vi "Configure Frequency Channel.vi"(7 "Enable Frequency Channel (F:Disable)":bool, 8 "error in (no error)":errorcluster, 9 "Channel Number (1)":i32=1, 10 "Channel Band (2: P-GSM Base)":u16(ring)=2 items=["NADC Base", "NADC Mobile", "P-GSM Base", "P-GSM Mobile", "E-GSM Base", "E-GSM Mobile", "R-GSM Base", "R-GSM Mobile", "DCS Base", "DCS Mobile", "PCS Base", "PCS Mobile", "GSM 450 Base", "GSM 450 Mobile", "GSM 480 Base", "GSM 480 Mobile", "GSM 850 Base", "GSM 850 Mobile", "800MHZ Base", "800MHZ Mobile", "1500MHZ Base", "1500MHZ Mobile", "Tetra Base 390/400", "Tetra Base 420/430", "Tetra Base 460/470", "Tetra Base 915/921", "Tetra Mobile 380/390", "Tetra Mobile 410/420", "Tetra Mobile 450/460", "Tetra Mobile 870/876", "PHS Standard", "DECT Standard"], 11 "VISA resource name":refnum<visa-resource-name>) -> (0 "error out":errorcluster, 3 "VISA resource name out":refnum<visa-resource-name>)   [LabVIEW 2014, in "Agilent PSG MXG Series.lvlib"]
doc: "Configures frequency channel and band.\n\n<B>Notes:</B>\n(1) This VI is valid only in E8247C, E8257C, E8267C, E8257D, E8267D, N5161A, N5162A, N5181A, N5182A, N5183A, N5171B, N5172B, N5181B, N5182B."
uses:
  Agilent PSG MXG Series.lvlib
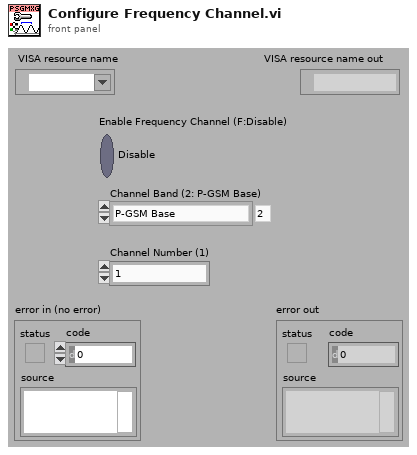
[diagram p1: front panel]
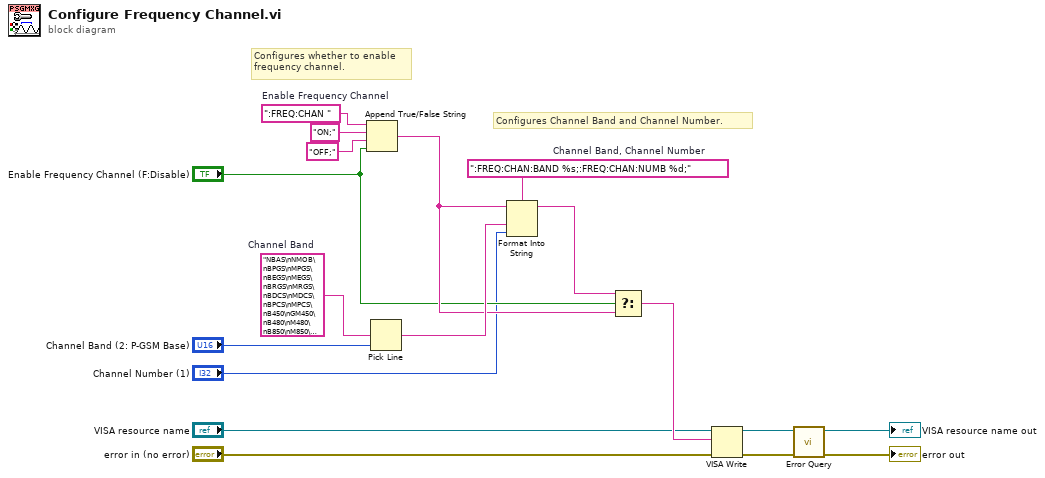
[diagram p0: block diagram]
diagram:
  w11 = ":FREQ:CHAN "  # Enable Frequency Channel
  w17 = ":FREQ:CHAN:BAND %s;:FREQ:CHAN:NUMB %d;"  # Channel Band, Channel Number
  w18 = "NBAS\nNMOB\nBPGS\nMPGS\nBEGS\nMEGS\nBRGS\nMRGS\nBDCS\nMDCS\nBPCS\nMPCS\nB450\nGM450\nB480\nM480\nB850\nM850\nB8\nM8\nB15\nM15\nB390\nB420\nB460\nB915\nM380\nM410\nM450\nM870\nPHS\nDECT"  # Channel Band
  # "Configures Channel Band and Channel Number."
  # "Configures whether to enable\nfrequency channel."
  n1 = Append True/False String(1:"Enable Frequency Channel (F:Disable)", 2:"OFF;" ("format string"), 3:"ON;" ("format string"), 4:w11) -> (0:w12:string)
  n2 = Pick Line(multi-line string=w18, line index="Channel Band (2: P-GSM Base)") -> (output string=w13:string)  [unwired: 1 out]
  n3 = Format Into String(format string=w17, initial string=w12, w13, "Channel Number (1)") -> (resulting string=w14:string)  [unwired: 1 in, 1 out]
  n4 = Select(t=w14, s="Enable Frequency Channel (F:Disable)", f=w12) -> (s? t:f=w5:string)
  n5 = VISA Write(VISA resource name="VISA resource name", write buffer=w5, error in (no error)="error in (no error)") -> (VISA resource name out=w7:refnum<visa-resource-name>, error out=w6:errorcluster)  [unwired: 1 out]
  n6 = call "Error Query.vi"("error in (no error)"=w6, "VISA resource name"=w7) -> ("error out"=→"error out":errorcluster, "VISA resource name out"=→"VISA resource name out":refnum<visa-resource-name>)  [unwired: 8 out]
